vi "get_number_of_ROIs.vi"(8 "error in (no error)":errorcluster, 11 "TrajectoryDL121017Hopping in":refnum<class "TrajectoryDL121017Hopping.lvclass">) -> (0 "error out":errorcluster, 2 "number of ROIs":i32, 3 "TrajectoryDL121017Hopping out":refnum<class "TrajectoryDL121017Hopping.lvclass">)   [LabVIEW 2010, in "TrajectoryDL121017Hopping.lvclass"]
doc: "Returns the number of uncaging ROIs."
uses:
  TrajectoryDL121017Hopping.lvclass
  TrajectoryDL121017Hopping.lvclass/TrajectoryDL121017Hopping.ctl
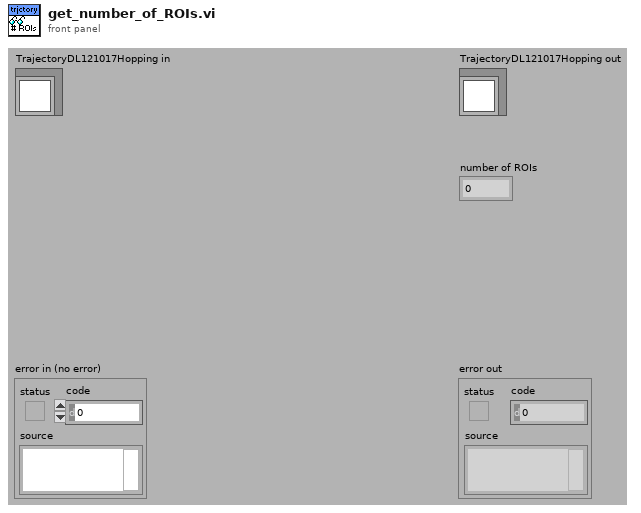
[diagram p1: front panel]
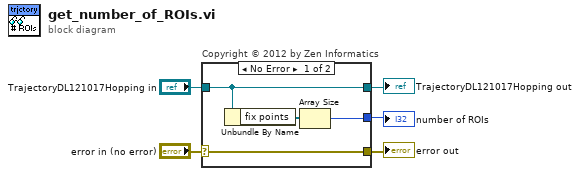
[diagram p0: block diagram]
diagram:
  n1 = case "Copyright © 2012 by Zen Informatics" shown="No Error" "error in (no error)" {
    selector: "error in (no error)" -> [w9 w11]
    tunnel: [w9 w11] -> w4
    tunnel: [w7 w10] -> w2
    tunnel: "TrajectoryDL121017Hopping in" -> [w7 w10]
    tunnel: [w6 _] -> w1
    frame No Error {
      n2 = Unbundle By Name(w7) -> ("fix points"=w8:refnum<class "SpaceVector.lvclass">[])
      n3 = Array Size(array=w8) -> (size(s)=w6:i32)
    }
    frame Error {
    }
  }
  "error out" <- w4
  "TrajectoryDL121017Hopping out" <- w2
  "number of ROIs" <- w1
